vi "PV OnTool Monitoring Operating Pumpsystem.vi"(8 "error in (no error)":errorcluster, 9 "PV OnTool Monitoring Op - Cluster":T1={"Parameter"=0, "Parameter\nread only<->describe"=FALSE, "Softpumping\nswitching\nthreshhold [hPa]"=267, "Soft pump rotation\nspeed in % of the\nfinal rpm [%]"=15, "Lower exhaust\ngas temperature\nlimit [C] "=5, "Upper exhaust\ngas temperature\nlimit [C]  "=250, "End of measuring\nrange of gauge"=0} {"End of measuring\nrange of gauge" items=[" 10 hPa", " 100 hPa", " 1000 hPa"]; "Upper exhaust\ngas temperature\nlimit [C]" min=5 max=280 step=1; "Lower exhaust\ngas temperature\nlimit [C]" min=5 max=200 step=1; "Soft pump rotation\nspeed in % of the\nfinal rpm [%]" min=15 max=100 step=1; "Softpumping\nswitching\nthreshhold [hPa]" min=0 max=1000 step=1; "Parameter" items=[" End of measuring range of gauge", " Exhaust pressure  [h/Pa]  (read only)", " Intake pressure  [hPa]  (read only)", " Temperature of pump housing [°C]   (read only)", " Motor temperature pump [°C] (read only)", " Temperature of exhaust gas [°C]   (read only)", " Softpumping switching threshhold [hPa]", " Soft pump rotation speed in % of the final rpm [%]", " Lower exhaust gas temperature limit [C]  ", " Upper exhaust gas temperature limit [C] "]}, 10 "Adress of unit":u16=1 max=999 step=1, 11 "VISA session":refnum<visa-resource-name>) -> (0 "error out":errorcluster, 2 "response (data)":string, 3 "dup VISA session":refnum<visa-resource-name>)   [LabVIEW 2016, in "Pfeiffer Vacuum.lvlib"]
doc: "There are 10 parameters available, only one of which can be enabled at a time. \n\n0 -End of measuring range of gauge (default) (Para.016)\n1 - Exhaust pressure [h/Pa] (read only) (Para.338)\n2 - Intake pressure [hPa] (read only) (Para.339)\n3 - Temperature of pump housing [°C] (read only) (Para.342)\n4 - Motor temperature pump [°C] (read only) (Para.346)\n5 - Temperature of exhaust gas [°C] (read only) (Para.343)\n6 - Softpumping switching threshhold [hPa] (Para.713)\n7 - Soft pump rotation speed in % of the final rpm [%] (Para.714) \n8 - Lower exhaust gas temperature limit [C] (Para.715) \n9 - Upper exhaust gas temperature limit [C] (Para.716)\n\nNote: The 5 controls right of this one will set the appropriate values for the selected parameter. Any settings for an parameter that is not selected will be ignored. If a value is out of range, it will be changed to either the upper or the lower limit of the range."
uses:
  Pfeiffer Vacuum.lvlib
  PV OnTool Monitoring Op - Cluster.ctl
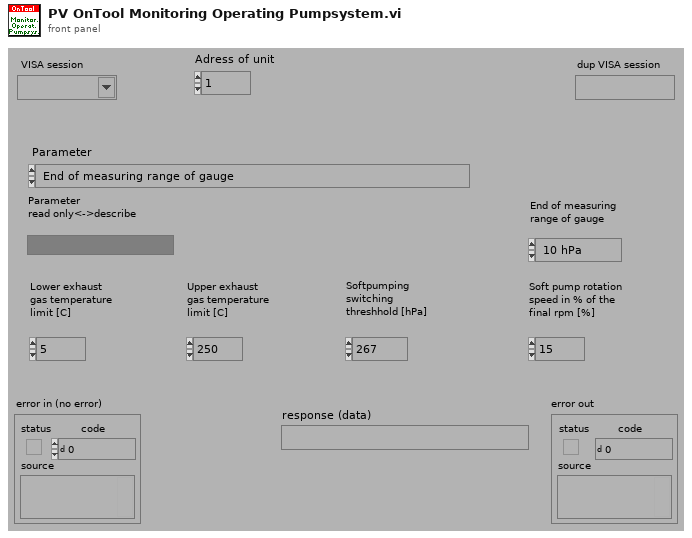
[diagram p1: front panel]
types:
  T1 = typedef "Pfeiffer Vacuum.lvlib/PV OnTool Monitoring Op - Cluster.ctl" = cluster{"Parameter":u16, "Parameter\nread only<->describe":bool, "Softpumping\nswitching\nthreshhold [hPa]":i16, "Soft pump rotation\nspeed in % of the\nfinal rpm [%]":u16, "Lower exhaust\ngas temperature\nlimit [C] ":u16, "Upper exhaust\ngas temperature\nlimit [C]  ":u16, "End of measuring\nrange of gauge":u16}
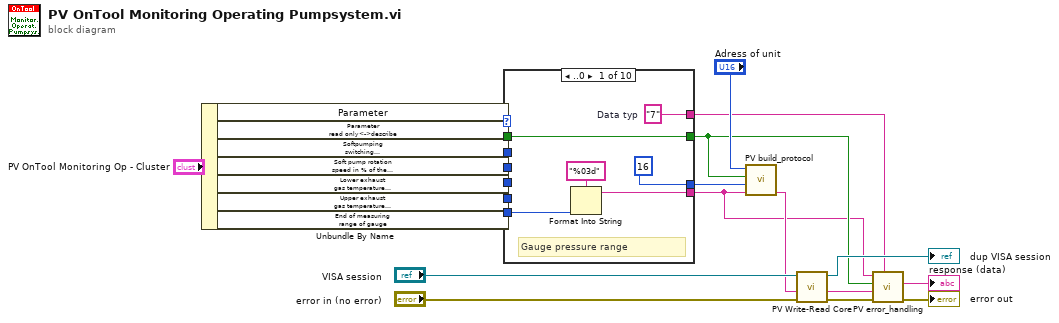
[diagram p0: block diagram]
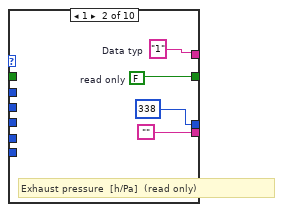
[diagram p2: hidden frame]
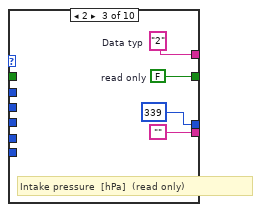
[diagram p3: hidden frame]
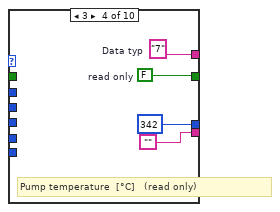
[diagram p4: hidden frame]
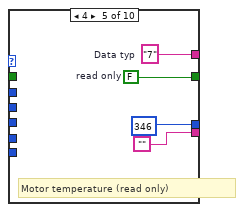
[diagram p5: hidden frame]
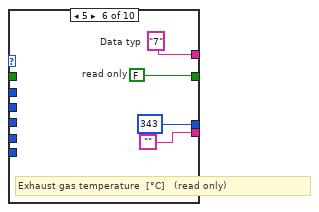
[diagram p6: hidden frame]
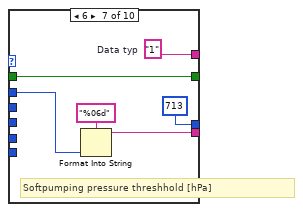
[diagram p7: hidden frame]
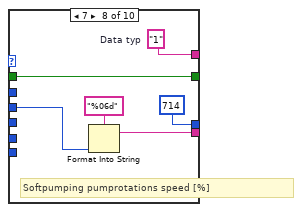
[diagram p8: hidden frame]
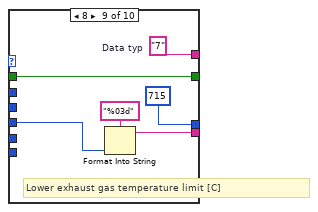
[diagram p9: hidden frame]
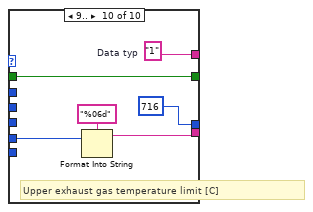
[diagram p10: hidden frame]
diagram:
  n1 = Unbundle By Name("PV OnTool Monitoring Op - Cluster") -> ("Parameter"=w18:u16, "Parameter\nread only<->describe"=w17:bool, "Softpumping\nswitching\nthreshhold [hPa]"=w16:i16, "Soft pump rotation\nspeed in % of the\nfinal rpm [%]"=w15:u16, "Lower exhaust\ngas temperature\nlimit [C]"=w14:u16, "Upper exhaust\ngas temperature\nlimit [C]"=w13:u16, "End of measuring\nrange of gauge"=w12:u16)
  n2 = case shown="..0" w18 {
    tunnel: [u16 16 ("Parameter-number") u16 338 ("Parameter-number") u16 339 ("Parameter-number") u16 342 ("Parameter-number") u16 346 ("Parameter-number") u16 343 ("Parameter-number") u16 713 ("Parameter-number") u16 714 ("Parameter-number") u16 715 ("Parameter-number") u16 716 ("Parameter-number")] -> w20
    tunnel: [w24 "" "" "" "" "" w50 w57 w65 w68] -> w4
    tunnel: [w26 w29 w33 w38 w43 w46 w52 w55 w62 w70] -> w5
    tunnel: w17 -> [w26 _ _ _ _ _ w52 w55 w62 w70]
    tunnel: w16 -> [_ _ _ _ _ _ w49 _ _ _]
    tunnel: w15 -> [_ _ _ _ _ _ _ w56 _ _]
    tunnel: w14 -> [_ _ _ _ _ _ _ _ w61 _]
    tunnel: w13 -> [_ _ _ _ _ _ _ _ _ w67]
    tunnel: w12 -> [w23 _ _ _ _ _ _ _ _ _]
    tunnel: [w22 w28 w32 w36 w42 w44 w48 w54 w60 w66] -> w3
    frame ..0 {
      w22 = "7"  # Data typ
      # "Gauge pressure range"
      n3 = Format Into String(format string="%03d" ("Format-String"), w23) -> (resulting string=w24:string)  [unwired: 2 in, 1 out]
    }
    frame 1 {
      w28 = "1"  # Data typ
      w29 = FALSE  # read only
      # "Exhaust pressure  [h/Pa]  (read only)"
    }
    frame 2 {
      w32 = "2"  # Data typ
      w33 = FALSE  # read only
      # "Intake pressure  [hPa]  (read only)"
    }
    frame 3 {
      w36 = "7"  # Data typ
      w38 = FALSE  # read only
      # "Pump temperature  [°C]   (read only)"
    }
    frame 4 {
      w42 = "7"  # Data typ
      w43 = FALSE  # read only
      # "Motor temperature (read only)"
    }
    frame 5 {
      w44 = "7"  # Data typ
      w46 = FALSE  # read only
      # "Exhaust gas temperature  [°C]   (read only)"
    }
    frame 6 {
      w48 = "1"  # Data typ
      # "Softpumping pressure threshhold [hPa]"
      n4 = Format Into String(format string="%06d" ("Format-String"), w49) -> (resulting string=w50:string)  [unwired: 2 in, 1 out]
    }
    frame 7 {
      w54 = "1"  # Data typ
      # "Softpumping pumprotations speed [%]"
      n5 = Format Into String(format string="%06d" ("Format-String"), w56) -> (resulting string=w57:string)  [unwired: 2 in, 1 out]
    }
    frame 8 {
      w60 = "7"  # Data typ
      # "Lower exhaust gas temperature limit [C]"
      n6 = Format Into String(format string="%03d" ("Format-String"), w61) -> (resulting string=w65:string)  [unwired: 2 in, 1 out]
    }
    frame 9.. {
      w66 = "1"  # Data typ
      # "Upper exhaust gas temperature limit [C]"
      n7 = Format Into String(format string="%06d" ("Format-String"), w67) -> (resulting string=w68:string)  [unwired: 2 in, 1 out]
    }
  }
  n8 = call "PV build_protocol.vi"("Data"=w4, "Parameter-number"=w20, "parameter\nread<->describe"=w5, "Adress"="Adress of unit") -> ("output"=w9:string)  [unwired: 3 in]
  n9 = call "PV Write-Read Core.vi"("error in"="error in (no error)", "Write data in"=w9, "VISA session"="VISA session") -> ("error out"=w6:errorcluster, "response (data) out"=w7:string, "dup VISA session"=→"dup VISA session":refnum<visa-resource-name>)  [unwired: 2 in]
  n10 = call "PV error_handling.vi"("Data Typ in"=w3, "error in"=w6, "response (data) in"=w7, "Parameter\nread only<->describe"=w5, "data in"=w4) -> ("error out"=→"error out":errorcluster, "Data out"=→"response (data)":string)  [unwired: 4 in, 1 out]
